vi "Match Names.vi"(8 "error in (no error)":errorcluster, 9 "Canonical":string, 10 "Alias":string, 11 "Driver in":refnum<class "Driver.lvclass">) -> (0 "error out":errorcluster, 2 "Recognised":bool, 3 "Driver out":refnum<class "Driver.lvclass">)   [LabVIEW 2023, in "HAF.lvlib" / "Driver.lvclass"]
doc: "Returns True if the Driver recognises either of the names passed."
uses:
  Driver.lvclass
  Driver.lvclass/Driver.ctl
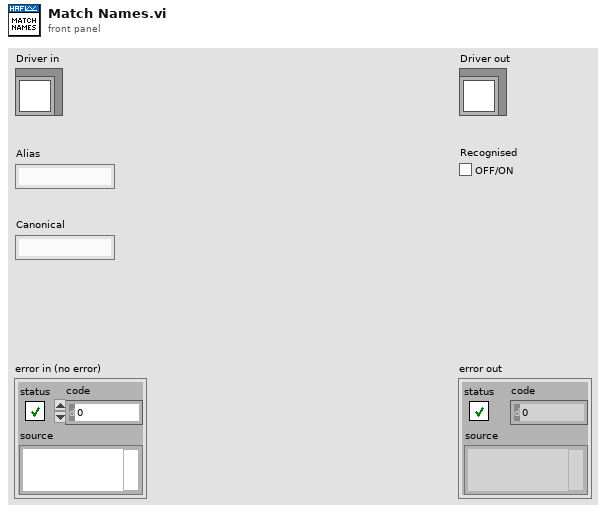
[diagram p1: front panel]
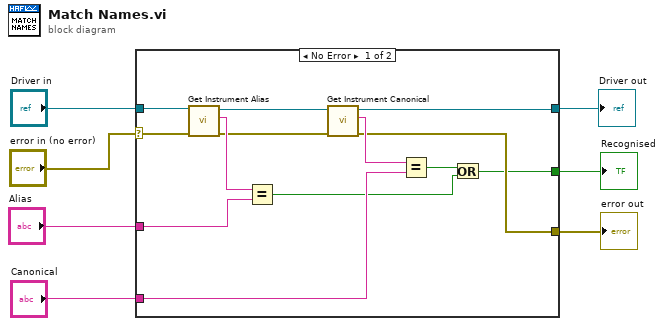
[diagram p0: block diagram]
diagram:
  n1 = case shown="No Error" "error in (no error)" {
    selector: "error in (no error)" -> [w19 w22]
    tunnel: [w10 w22] -> w6
    tunnel: [w8 w21] -> w4
    tunnel: "Driver in" -> [w20 w21]
    tunnel: "Alias" -> [w17 _]
    tunnel: "Canonical" -> [w13 _]
    tunnel: [w9 _] -> w1
    frame No Error {
      n2 = call-dynamic "Get Instrument Alias.vi"("error in (no error)"=w19, "Driver in"=w20) -> ("error out"=w15:errorcluster, "Instrument Alias"=w18:string, "Driver out"=w16:refnum<class "Driver.lvclass">)  [unwired: 7 in]
      n3 = Equal?(x=w18, y=w17) -> (x = y?=w11:bool)
      n4 = call-dynamic "Get Instrument Canonical.vi"("error in (no error)"=w15, "Driver in"=w16) -> ("error out"=w10:errorcluster, "Canonical Name"=w14:string, "Driver out"=w8:refnum<class "Driver.lvclass">)  [unwired: 7 in]
      n5 = Equal?(x=w14, y=w13) -> (x = y?=w12:bool)
      n6 = Or(x=w12, y=w11) -> (x .or. y?=w9:bool)
    }
    frame Error {
    }
  }
  "error out" <- w6
  "Driver out" <- w4
  "Recognised" <- w1
